vi "SVT Frequency Response Subset (Mag-Phase).vi"(0 "stimulus signal X [EUx]":waveform(dbl)={"t0"=timestamp(0 s since 1904-01-01), "dt"=1e-05, "Y"=[]}, 1 "response signal Y [EUy]":waveform(dbl)={"t0"=timestamp(0 s since 1904-01-01), "dt"=1e-05, "Y"=[]}, 2 "window":T9=1 items=["None"=0, "Hanning"=1, "Hamming"=2, "Blackman-Harris"=3, "Exact Blackman"=4, "Blackman"=5, "Flat Top"=6, "4 Term B-Harris "=7, "7 Term B-Harris"=8, "Low Sidelobe"=9, "Force - Exponential"=10, "Blackman Nuttall"=11, "Triangle"=30, "Bartlett-Hanning"=31, "Bohman"=32, "Parzen"=33, "Welch"=34, "Kaiser"=60, "Dolph-Chebyshev"=61, "Gaussian"=62], 3 "frequency range":T7={"start frequency"=1000.0, "stop frequency"=5000.0} {"stop frequency" min=0.0 format="%.2f"; "start frequency" min=0.0 format="%.2f"}, 4 "view":T11={"dB On (T)"=TRUE, "unwrap phase (F)"=FALSE, "convert to degree (T)"=TRUE}, 5 "error in (no error)":errorcluster, 6 "FRF mode":enum16{"H1", "H2", "H3"}(ring), 7 "averaging parameters":T10={"averaging mode"=enum."No averaging", "weighting mode"=enum."Exponential", "number of averages"=10, "linear mode"=enum."One shot"}, 8 "force/exp settings":T8={"force window [%]"=50.0, "exp window [%]"=10.0} {"exp window [%]" min=0.0 max=100.0 format="%.2f"; "force window [%]" min=0.0 max=100.0 format="%.2f"}, 9 "restart averaging (F)":bool) -> (11 "averaging done":bool, 12 "coherence":cluster{"f0":dbl, "df":dbl, "coherence":dbl[]}={"f0"=nan, "df"=inf, "coherence"=[]} {"coherence" format="%.2f"; "df" format="%.2f"; "f0" format="%.2f"}, 13 "averages completed":dbl, 14 "magnitude [dB EUy/EUx]":cluster{"f0":dbl, "df":dbl, "magnitude":dbl[]}={"f0"=nan, "df"=inf, "magnitude"=[]} {"magnitude" format="%.2f"; "df" format="%.2f"; "f0" format="%.2f"}, 15 "magnitude unit label":string="dB rms ref 1.0E+0 ", 16 "phase [degrees]":cluster{"f0":dbl, "df":dbl, "phase":dbl[]}={"f0"=nan, "df"=inf, "phase"=[]} {"phase" format="%.2f"; "df" format="%.2f"; "f0" format="%.2f"}, 17 "phase unit label":string="degree", 18 "spectrum info":T1={"channel name"="", "description"="", "x-axis units"=1, "spectral info"={"spectrum type"=enum."Power [Magnitude^2]", "linear/dB"=enum."linear", "window"=0, "window size"=0, "FFT size"=0}, "engineering units"=0, "custom label"="", "dB reference [EU]"=0.0, "peak units"=enum."rms", "weighting filter"=0, "spectral density?"=FALSE, "unit label"="", "spectrum skewed?"=FALSE, "complimentary spectrum units"=enum."none"} {"x-axis units" items=["Time (s)"=0, "Frequency-CB (Hz)"=1, "Frequency-CPB (Hz)"=1248, "Frequency-Arbitrary (Hz)"=2357, "Quefrency (s)"=2, "Revolutions (rev)"=3, "Order"=4, "Speed (RPM)"=11, "Speed (rad/s)"=21, "Index"=65535]; "weighting filter" items=["Linear", "A-weighting", "B-weighting", "C-weighting", "ITU-R 468-4", "Dolby", "CCITT", "C-message", "Wb", "Wc", "Wd", "We", "Wf", "Wh", "Wj", "Wk", "Wm", "AES17 20 kHz lowpass", "AES17 40 kHz lowpass", "AES17 20 kHz highpass", "AES17 40 kHz highpass"]; "dB reference [EU]" format="%.2f"; "engineering units" items=["custom..."=0, "V"=1, "A"=21, "C"=30, "pC"=31, "s"=32, "-"=29, "Pa"=2, "N"=20, "g"=3, "m/s^2"=4, "m/s"=5, "m"=6, "mm/s"=12, "mm"=13, "micron/s"=14, "micron"=15, "in/s^2"=7, "in/s"=8, "in"=9, "mil/s"=10, "mil"=11, "rad/s^2"=16, "rad/s"=17, "rad"=18, "deg/s^2"=26, "deg/s"=27, "deg"=28, "RPM"=22, "cycle/s^2"=23, "Hz"=24, "cycle"=25, "strain"=19]; "spectral info"."window" items=["None "=0, "Hanning"=1, "Hamming"=2, "Blackman-Harris"=3, "Exact Blackman"=4, "Blackman"=5, "Flat Top"=6, "4 Term B-Harris "=7, "7 Term B-Harris"=8, "Low Sidelobe"=9, "Force - Exponential"=10, "Gaussian"=62]}, 19 "error out":errorcluster)   [LabVIEW 2017]
doc: "Computes a subset of the frequency response and of the coherence based on <B>stimulus signal X [EUx]</B> and <B>response signal Y [EUy]</B>. The subset is defined by <B>frequency range</B>. Results are returned in <B>coherence</B>, <B>magnitude [dB EUy/EUx]</B>, and <B>phase [degrees]</B>."
uses:
  <vilib>/addons/_NISVFA/_Shared subVIs/Controls/svc_Window [Dual FFT].ctl
  <vilib>/addons/_NISVFA/_Shared subVIs/Controls/svc_Spectrum Info.ctl
  <vilib>/addons/_NISVFA/_Shared subVIs/Controls/svc_X-Axis Units.ctl
  <vilib>/addons/_NISVFA/_Shared subVIs/Controls/svc_Spectrum Type.ctl
  <vilib>/addons/_NISVFA/_Shared subVIs/Controls/svc_Engineering Units Text Ring.ctl
  <vilib>/addons/_NISVFA/_Shared subVIs/Controls/svc_Weighting Filter Text Ring.ctl
  <vilib>/addons/_NISVFA/_Shared subVIs/Controls/svc_Complimentary Spectrum Units.ctl
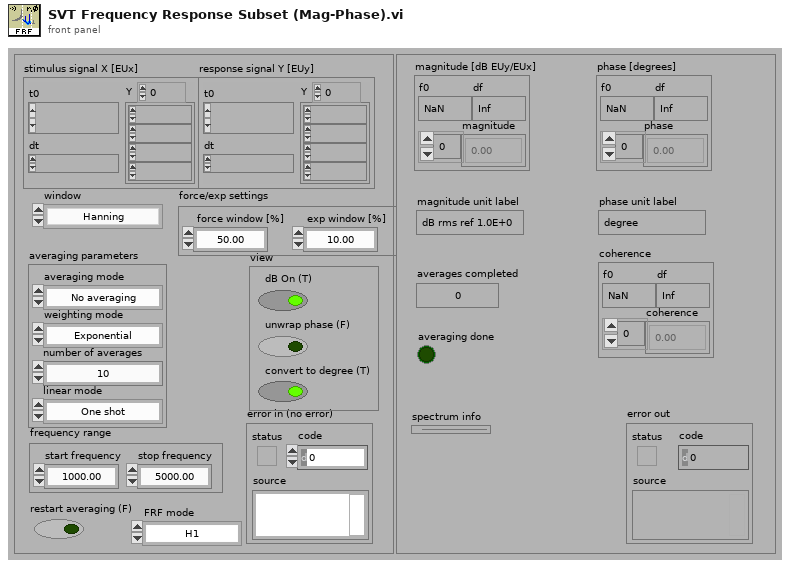
[diagram p1: front panel]
types:
  T1 = typedef "svc_Spectrum Info.ctl" = cluster{"channel name":string, "description":string, "x-axis units":T2, "spectral info":cluster{"spectrum type":T3, "linear/dB":enum16{"linear", "dB"}, "window":u16, "window size":i32, "FFT size":i32}, "engineering units":T4, "custom label":string, "dB reference [EU]":dbl, "peak units":enum16{"rms", "peak", "peak-peak"}, "weighting filter":T5, "spectral density?":bool, "unit label":string, "spectrum skewed?":bool, "complimentary spectrum units":T6}
  T2 = typedef "svc_X-Axis Units.ctl" = u16
  T3 = typedef "svc_Spectrum Type.ctl" = enum16{"FFT Spectrum [complex]", "Amplitude [Magnitude]", "Power [Magnitude^2]", "Cross Spectrum [complex]", "Frequency Response [Complex]"}
  T4 = typedef "svc_Engineering Units Text Ring.ctl" = u16
  T5 = typedef "svc_Weighting Filter Text Ring.ctl" = u16
  T6 = typedef "svc_Complimentary Spectrum Units.ctl" = enum16{"none", "radians", "degrees", "cycles", "imaginary"}
  T7 = cluster{"start frequency":dbl, "stop frequency":dbl}
  T8 = cluster{"force window [%]":dbl, "exp window [%]":dbl}
  T9 = typedef "svc_Window [Dual FFT].ctl" = u32
  T10 = cluster{"averaging mode":enum16{"No averaging", "Vector averaging", "RMS averaging", "Peak hold"}, "weighting mode":enum16{"Linear", "Exponential"}, "number of averages":u32, "linear mode":enum16{"One shot", "Auto restart"}}
  T11 = cluster{"dB On (T)":bool, "unwrap phase (F)":bool, "convert to degree (T)":bool}
  T12 = enum16{"Cross spectrum", "Frequency response", "Coherent output power"}
  T13 = enum16{"Restart processing", "Continue processing", "Skip processing"}
  T14 = cluster{"f0":dbl, "df":dbl, "complex spectrum":cdb[]}
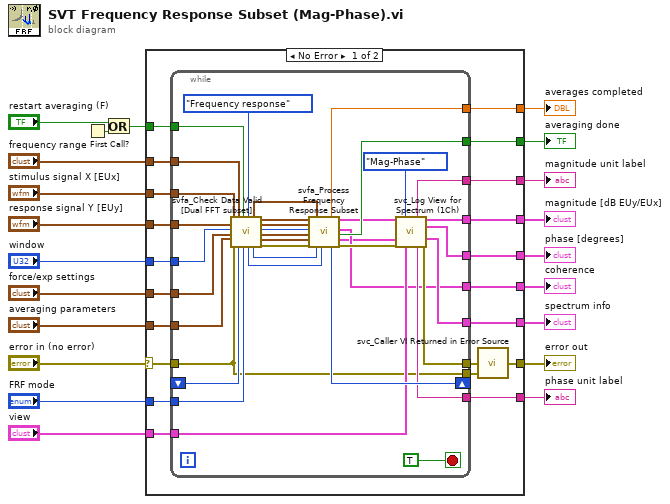
[diagram p0: block diagram]
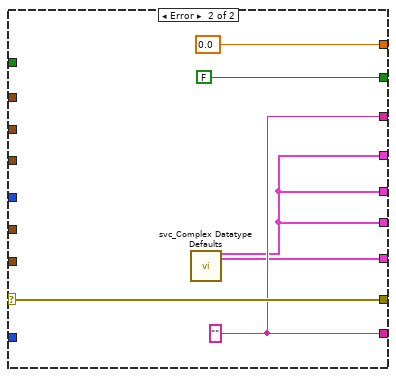
[diagram p2: hidden frame]
diagram:
  n1 = First Call?() -> (First Call?: T/F=w3:bool)
  n2 = Or(x="restart averaging (F)", y=w3) -> (x .or. y?=w1:bool)
  n3 = case shown="No Error" "error in (no error)" {
    selector: "error in (no error)" -> [w35 w84]
    tunnel: "averaging parameters" -> [w36 _]
    tunnel: "window" -> [w38 _]
    tunnel: "force/exp settings" -> [w37 _]
    tunnel: "stimulus signal X [EUx]" -> [w42 _]
    tunnel: "response signal Y [EUy]" -> [w39 _]
    tunnel: [w30 w79] -> w15
    tunnel: [w29 w79] -> w14
    tunnel: [w28 w79] -> w13
    tunnel: [w23 w84] -> w12
    tunnel: [w32 0.0 ("averages completed")] -> w11
    tunnel: w1 -> [w40 _]
    tunnel: "view" -> [w25 _]
    tunnel: "frequency range" -> [w41 _]
    tunnel: [w34 FALSE ("averaging done")] -> w8
    tunnel: "FRF mode" -> [w33 _]
    tunnel: [w31 w81] -> w6
    tunnel: [w27 w80] -> w5
    tunnel: [w24 w81] -> w4
    frame No Error {
      n4 = while {
        tunnel: [w49] -> w24
        tunnel: w25 -> [w50]
        tunnel: [w51] -> w26
        tunnel: [w52] -> w27
        tunnel: [w45] -> w28
        tunnel: [w46] -> w29
        tunnel: [w53] -> w30
        tunnel: [w54] -> w31
        tunnel: [w55] -> w32
        tunnel: w33 -> [w58]
        tunnel: [w64] -> w34
        tunnel: w35 -> [w43]
        tunnel: w36 -> [w71]
        tunnel: w37 -> [w72]
        tunnel: w38 -> [w73]
        tunnel: w39 -> [w74]
        tunnel: w40 -> [w75]
        tunnel: w41 -> [w76]
        tunnel: w42 -> [w77]
        shift-left: _ -> [w61]
        shift-right: [w59] -> _
        tunnel: [w43] -> w22
        stop <- TRUE stop-if-true
        n5 = call <vilib>:"svfa_Check Data Valid [Dual FFT subset].vi"("stimulus [X]"=w77, "response [Y]"=w74, "window"=w73, "force/exp settings"=w72, "averaging parameters"=w71, "error in (no error)"=w43, "frequency range"=w76, "processing control in"=w61, "restart averaging (F)"=w75, "FRF mode"=w58, "measurement"=T12."Frequency response") -> ("dup FRF mode"=w57:enum16{"H1", "H2", "H3"}, "dup frequency range"=w56:T7, "processing control out"=w60:T13, "dup stimulus [X]"=w70:waveform(dbl), "dup response [Y]"=w69:waveform(dbl), "window"=w68:u16, "dup force/exp settings"=w67:T8, "dup averaging parameters"=w66:T10, "error out"=w65:errorcluster)
        n6 = call <vilib>:"svfa_Process Frequency Response Subset.vi"("Windowed signal [X]"=w70, "Windowed signal [Y]"=w69, "window (includes Force_Exp)"=w68, "force/exp settings"=w67, "averaging parameters"=w66, "error in (no error)"=w65, "Spectrum Settings"=w56, "processing control"=w60, "FRF mode"=w57) -> ("averages completed"=w55:dbl, "processing control"=w59:T13, "complex frequency response"=w63:T14, "Coherence"=w45:cluster{"f0":dbl, "df":dbl, "Spectrum":dbl[]}, "averaging done"=w64:bool, "spectrum info"=w44:T1, "error out"=w47:errorcluster)  [unwired: 4 in]
        n7 = call <vilib>:"svc_Log View for Spectrum (1Ch).vi"("complex spectrum"=w63, "View"=enum16{"Mag-Phase", "Real-Imaginary"}."Mag-Phase", "spectrum info in"=w44, "error in (no error)"=w47, "view"=w50) -> ("unit label [mag or real]"=w54:string, "magnitude or real"=w53:cluster{"f0":dbl, "df":dbl, dbl[]}, "phase or imag"=w46:cluster{"f0":dbl, "df":dbl, dbl[]}, "spectrum info out"=w52:T1, "unit label [phase or imag]"=w49:string, "error out"=w51:errorcluster)  [unwired: 5 in]
      }
      n8 = call <vilib>:"svc_Caller VI Returned in Error Source.vi"("warning input to caller"=w22, "error in (no error)"=w26) -> ("error out"=w23:errorcluster)  [unwired: 3 in]
    }
    frame Error {
      w81 = "" ("unit label (mag or real)")
      n9 = call <vilib>:"svc_Complex Datatype Defaults.vi"() -> ("empty spectrum"=w79:cluster{"f0":dbl, "df":dbl, "magnitude":dbl[]}, "dead spectrum info"=w80:T1)  [unwired: 11 in, 7 out]
    }
  }
  "error out" <- w12
  "magnitude [dB EUy/EUx]" <- w15
  "phase [degrees]" <- w14
  "averaging done" <- w8
  "averages completed" <- w11
  "coherence" <- w13
  "spectrum info" <- w5
  "magnitude unit label" <- w6
  "phase unit label" <- w4
